vi "AR Example Master.vi"() -> ()   [LabVIEW 2020]
uses:
  UI_Actor/UI_Actor/ctl_AR_Parameters.ctl
  UI_Actor/UI_Actor/ctl_AR_Mode.ctl
  UIA_ChildTestMaster/UIA_ChildTestMaster.lvclass
  D:/Projets/STEP AT/UI Actor/UI_Actor/UI_Actor/UI_Actor.lvclass
  UI_Actor/UI_Actor Messages/UI_ShowIn_FreeWindow Msg/UI_ShowIn_FreeWindow Msg.lvclass/UI_ShowIn_FreeWindow Msg.ctl
  support/Databox.lvlibp/TypesTools/Config/Config.lvclass
  support/Databox.lvlibp/TypesTools/Data/Data.lvclass
  support/Databox.lvlibp/TypesTools/Data/TypeEnum.ctl
  UI_Actor/UI_Actor Messages/UI_AutoRefresh Msg/UI_AutoRefresh Msg.lvclass/UI_AutoRefresh Msg.ctl
  support/Actor Framework.lvlibp/1abvi3w/vi.lib/ActorFramework/Message Enqueuer/Enqueue.vi
  UI_Actor/UI_Actor Messages/UI_ShowIn_FreeWindow Msg/UI_ShowIn_FreeWindow Msg.lvclass
  UI_Actor/UI_Actor Messages/UI_AutoRefresh Msg/UI_AutoRefresh Msg.lvclass
  UI_Actor/UI_Actor/UI_Actor.lvclass
  support/Actor Framework.lvlibp/1abvi3w/vi.lib/ActorFramework/Stop Msg/Stop Msg.lvclass
panel:
  in  "Data 2":dbl[](array[numeric])=[0.0, 0.0]
  in  "Units 2":string[](array[string])=["ppm", "sec"]
  in  "UserLab 2":string[](array[string])=["", "0"]
  in  "SysLab 2":string[](array[string])=["indic", "Time"]
  in  "Data":dbl[](array[numeric])=[2.0, 2.0, 5.0, 0.0, 0.0, 0.0, 0.0, 3.0, 0.0]
  in  "Parameters":T1={"Write TipStrips with details (T)"=TRUE, "Write Captions with UserLabels (T)"=TRUE, "Mode (ind only)"=enum."All"}
  in  "Units":string[](array[string])=["%", "km", "°C", "-", "", "", " ", "kV", "A"]
  in  "UserLab":string[](array[string])=["coucou 1", "coucou 2", "temp", "c chaud", "", "", " ", "yes!", "Clust num"]
  in  "SysLab":string[](array[string])=["Ctl1", "Ctl2", "indic1", "indic2", "ring", "enum", "slide", "Indic3 in tab ctl", "Clust num"]
  in  "stop":bool
  # "MASTER            --- launches ->    SUB\nrank 0                                               rank 1"
  # "Sourcer: S1"
  # "Sourcer: S2"
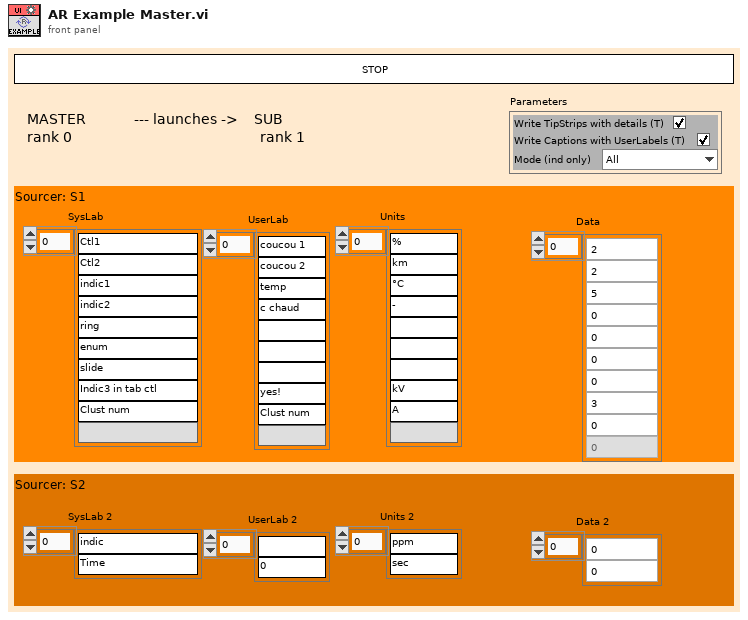
[diagram p1: front panel]
types:
  T1 = typedef "UI_Actor.lvlib/UI_Actor.lvclass/ctl_AR_Parameters.ctl" = cluster{"Write TipStrips with details (T)":bool, "Write Captions with UserLabels (T)":bool, "Mode (ind only)":T2}
  T2 = typedef "UI_Actor.lvlib/UI_Actor.lvclass/ctl_AR_Mode.ctl" = enum16{"Controls only", "Indicators only", "All"}
  T3 = cluster{"Ch.Conf":refnum<class "Config.lvclass">, "Data":refnum<class "Data.lvclass">[]}
  T4 = typedef "Databox.lvlibp/Data.lvclass/TypeEnum.ctl" = enum16{"Boolean", "SByte", "Byte", "Int16", "UInt16", "Int32", "UInt32", "Int64", "UInt64", "Float", "Double", "String", "DateTime", "ByteString", "Array of Boolean", "Array of SByte", "Array of Byte", "Array of Int16", "Array of UInt16", "Array of Int32", "Array of UInt32", "Array of Int64", "Array of UInt64", "Array of Float", "Array of Double", "Array of String", "Array of DateTime", "Array of ByteString", "Matrix of Boolean", "Matrix of SByte", "Matrix of Byte", "Matrix of Int16", "Matrix of UInt16", "Matrix of Int32", "Matrix of UInt32", "Matrix of Int64", "Matrix of UInt64", "Matrix of Float", "Matrix of Double", "Matrix of String ", "Matrix of DateTime", "Matrix of ByteString"}
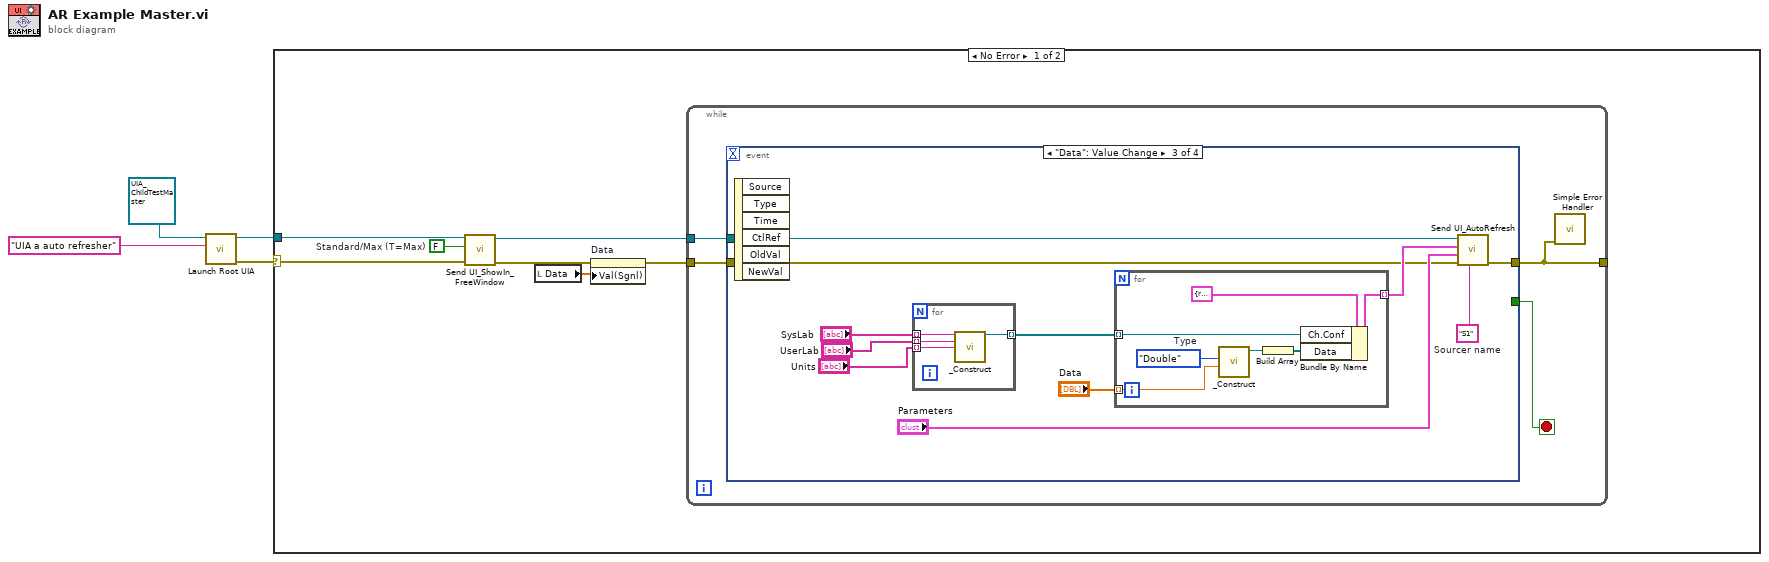
[diagram p0: block diagram]
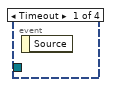
[diagram p2: hidden frame]
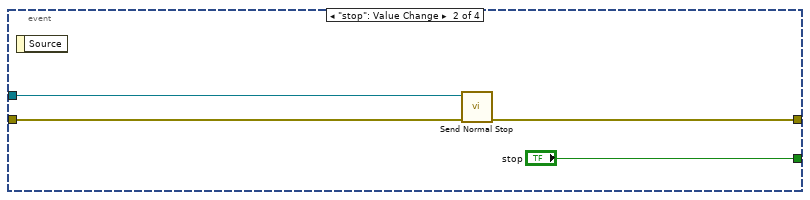
[diagram p3: hidden frame]
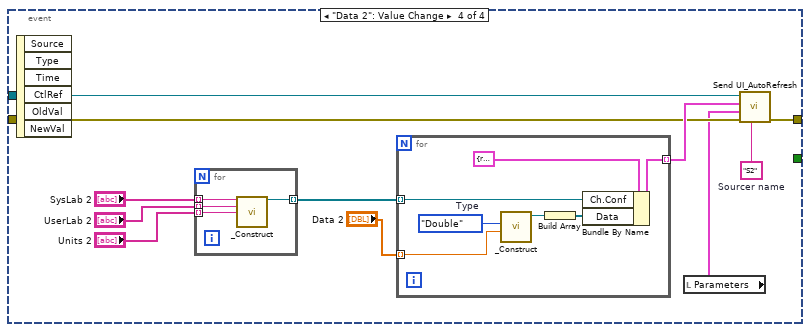
[diagram p4: hidden frame]
diagram:
  n1 = call "Launch Root UIA.vi"("Actor Name"="UIA a auto refresher", "UI_Actor in"=refnum<class "UIA_ChildTestMaster.lvclass"> refnum ("UIA_ChildTestMaster.lvclass")) -> ("error out"=w3:errorcluster, "Actor's Enqueuer"=w4:refnum<class "Message Enqueuer.lvclass">)  [unwired: 8 in]
  n2 = case shown="No Error" w3 {
    selector: w3 -> [w10 _]
    tunnel: w4 -> [w11 _]
    frame No Error {
      w8 = FALSE  # Standard/Max (T=Max)
      n3 = call "Send UI_ShowIn_FreeWindow.vi"("error in (no error)"=w10, "Standard/Max (T=Max)"=w8, "Message Enqueuer"=w11) -> ("error out"=w7:errorcluster, "Message Enqueuer out"=w9:refnum<class "Message Enqueuer.lvclass">)  [unwired: 7 in]
      n4 = local read "Data"() -> (w5:dbl[])
      n5 = property on="Data" class="Arr (strict)"(error in=w7, "Val(Sgnl)"=w5) -> (error out=w6:errorcluster)  [unwired: 1 in, 1 out]
      n6 = while {
        tunnel: w9 -> [w14]
        tunnel: [w12] -> _
        tunnel: w6 -> [w13]
        stop <- w15 stop-if-true
        n7 = event shown="[2] \"Data\": Value Change" {
          selector: _ -> [_ _ _ _]
          dyn-events: _ -> [_ _ _ _]
          timeout: _ -> [_ _ _ _]
          tunnel: [_ "stop" _ _] -> w15
          tunnel: w14 -> [_ w18 w27 w51]
          tunnel: [_ w16 w25 w49] -> w12
          tunnel: w13 -> [_ w17 w26 w50]
          event Timeout {
            n8 = event-data() -> ()  [unwired: 1 in, 1 out]
          }
          event "stop": Value Change {
            n9 = event-data() -> ()  [unwired: 1 in, 1 out]
            n10 = call "Send Normal Stop.vi"("error in (no error)"=w17, "Message Enqueuer"=w18) -> ("error out"=w16:errorcluster)  [unwired: 9 in]
          }
          event "Data": Value Change {
            w20 = "S1"  # Sourcer name
            n11 = event-data() -> ()  [unwired: 1 in, 6 out]
            n12 = for {
              tunnel: [w34] -> w21 mode=indexing
              tunnel: "SysLab" -> [w33] mode=indexing
              tunnel: "UserLab" -> [w32] mode=indexing
              tunnel: "Units" -> [w31] mode=indexing
              n13 = call "_Construct.vi"("System Label"=w33, "User Label"=w32, "Unit"=w31) -> ("Ch.Conf out"=w34:refnum<class "Config.lvclass">)  [unwired: 11 in, 1 out]
            }
            n14 = for {
              tunnel: [w40] -> w29 mode=indexing
              tunnel: w21 -> [w39] mode=indexing
              tunnel: "Data" -> [w35] mode=indexing
              w36 = TypeEnum."Double"  # Type
              n15 = call "_Construct.vi"("Value"=w35, "Type"=w36) -> ("Ch.TData out"=w38:refnum<class "Data.lvclass">)  [unwired: 8 in, 1 out]
              n16 = Build Array(w38) -> (w37:refnum<class "Data.lvclass">[])
              n17 = Bundle By Name(cluster=T3 {"Ch.Conf"=refnum, "Data"=[]} ("Cluster"), "Ch.Conf"=w39, "Data"=w37) -> (w40:T3)
            }
            n18 = call "Send UI_AutoRefresh.vi"("Sourcer name"=w20, "error in (no error)"=w26, "Parameters (Tipstrips,Captions,All)"="Parameters", "Data chunk"=w29, "Message Enqueuer"=w27) -> ("error out"=w25:errorcluster)  [unwired: 5 in, 1 out]
          }
          event "Data 2": Value Change {
            w43 = "S2"  # Sourcer name
            n19 = event-data() -> ()  [unwired: 1 in, 6 out]
            n20 = for {
              tunnel: [w56] -> w48 mode=indexing
              tunnel: "SysLab 2" -> [w55] mode=indexing
              tunnel: "UserLab 2" -> [w54] mode=indexing
              tunnel: "Units 2" -> [w53] mode=indexing
              n21 = call "_Construct.vi"("System Label"=w55, "User Label"=w54, "Unit"=w53) -> ("Ch.Conf out"=w56:refnum<class "Config.lvclass">)  [unwired: 11 in, 1 out]
            }
            n22 = for {
              tunnel: [w62] -> w52 mode=indexing
              tunnel: w48 -> [w61] mode=indexing
              tunnel: "Data 2" -> [w57] mode=indexing
              w58 = TypeEnum."Double"  # Type
              n23 = call "_Construct.vi"("Value"=w57, "Type"=w58) -> ("Ch.TData out"=w60:refnum<class "Data.lvclass">)  [unwired: 8 in, 1 out]
              n24 = Build Array(w60) -> (w59:refnum<class "Data.lvclass">[])
              n25 = Bundle By Name(cluster=T3 {"Ch.Conf"=refnum, "Data"=[]} ("Cluster"), "Ch.Conf"=w61, "Data"=w59) -> (w62:T3)
            }
            n26 = local read "Parameters"() -> (w42:T1)
            n27 = call "Send UI_AutoRefresh.vi"("Sourcer name"=w43, "error in (no error)"=w50, "Parameters (Tipstrips,Captions,All)"=w42, "Data chunk"=w52, "Message Enqueuer"=w51) -> ("error out"=w49:errorcluster)  [unwired: 5 in, 1 out]
          }
        }
        n28 = call <vilib>:"Simple Error Handler.vi"("error in (no error)"=w12) -> ()  [unwired: 4 in, 5 out]
      }
    }
    frame Error {
    }
  }
